vi "Version_2.0_Single_Column_Code.vi"() -> ()   [LabVIEW 2020] (continued)
                            n921 = local write "Valve V6 Open"(FALSE ("Valve V6 Open")) -> ()
                            n922 = local write "Valve V7 Open"(FALSE ("Valve V7 Open")) -> ()
                          }
                          frame #3 {
                            n923 = local read "Apparent Volume\nof Syringe"() -> (w1396:dbl)
                            n924 = local read "Sample Volume \nto be Pumped"() -> (w1399:dbl)
                            n925 = Quotient & Remainder(x=w1399, y=w1396) -> (x-y*floor(x/y)=w1397:dbl, floor(x/y)=w1398:dbl)
                            n926 = for {
                              N: w1398 -> [_]
                              n927 = stacked-sequence {
                                frame #0 {
                                n928 = local read "Sample PickUp \nFlow Rate (ul/min)"() -> (w1402:dbl)
                                n929 = local read "Sample Pumping\nResolution"() -> (w1401:T2)
                                n930 = local read "VISA Refnum in\nfor Pump"() -> (w1404:refnum<visa-resource-name>)
                                n931 = local read "Apparent Volume\nof Syringe"() -> (w1400:dbl)
                                n932 = local read "Volume of Syringe"() -> (w1403:dbl)
                                n933 = call "RPickUp(SubVI).vi"("Volume to be picked up"=w1400, "Volume of Syringe"=w1403, "Resolution of PickUP"=w1401, "PickUp Flow Rate (ul/min)"=w1402, "VISA Refnum in"=w1404) -> ()  [unwired: 6 in, 1 out]
                                }
                                frame #1 {
                                n934 = local read "Stopper that ends \nthe main loops"() -> (w1405:bool)
                                n935 = local read "VISA Refnum in\nfor Pump"() -> (w1406:refnum<visa-resource-name>)
                                n936 = case shown="True" w1405 {
                                frame False {
                                }
                                frame True {
                                n937 = local read "VISA Refnum in\nfor Pump"() -> (w1407:refnum<visa-resource-name>)
                                n938 = call "HardStopCurrentProcess (SubVI).vi"("VISA Refnum in"=w1407) -> ()  [unwired: 11 in]
                                }
                                }
                                n939 = call "ProcessCompletionWaiter (SubVI).vi"("VISA Refnum in"=w1406) -> ()  [unwired: 11 in]
                                }
                                frame #2 {
                                # "Reads the initial Plunger Position for computing the volume dispensed"
                                n940 = local read "VISA Refnum in\nfor Pump"() -> (w1409:refnum<visa-resource-name>)
                                n941 = call "AbsolutePlungerPosition (SubVI).vi"("VISA Refnum in"=w1409) -> ("Plunger Position"=w1408:i32)  [unwired: 10 in]
                                n942 = local write "Initial Plunger Position"(w1408) -> ()
                                }
                                frame #3 {
                                # "Switch to Port-2"
                                # "Port-2 of the pump is conncted to column-1 of chip"
                                n943 = local read "VISA Refnum in\nfor Pump"() -> (w1411:refnum<visa-resource-name>)
                                n944 = call "PortChanger (SubVI).vi"("Port Number"="2", "VISA Refnum in"=w1411) -> ()  [unwired: 10 in]
                                }
                                frame #4 {
                                n945 = local read "Stopper that ends \nthe main loops"() -> (w1412:bool)
                                n946 = local read "VISA Refnum in\nfor Pump"() -> (w1413:refnum<visa-resource-name>)
                                n947 = case shown="True" w1412 {
                                frame False {
                                }
                                frame True {
                                n948 = local read "VISA Refnum in\nfor Pump"() -> (w1414:refnum<visa-resource-name>)
                                n949 = call "HardStopCurrentProcess (SubVI).vi"("VISA Refnum in"=w1414) -> ()  [unwired: 11 in]
                                }
                                }
                                n950 = call "ProcessCompletionWaiter (SubVI).vi"("VISA Refnum in"=w1413) -> ()  [unwired: 11 in]
                                }
                                frame #5 {
                                # "Keeps the AMF valve after column-1 open and valve after column-2 closed"
                                n951 = local read "Sample Dispense\nFlow Rate (ul/min)"() -> (w1418:dbl)
                                n952 = local read "Sample Pumping\nResolution"() -> (w1417:T2)
                                n953 = local read "VISA Refnum in\nfor Pump"() -> (w1420:refnum<visa-resource-name>)
                                n954 = local write "Pause Data Collection"(FALSE ("Pause Data Collection")) -> ()
                                n955 = local read "Volume of Syringe"() -> (w1419:dbl)
                                n956 = call "GoToAbsolutePosition(SubVI).vi"("Absolute Volume Position in Syringe (in ul)"=0.0 ("Volume to be Dispensed"), "Volume of Syringe"=w1419, "Resolution of Pumping"=w1417, "Flow Rate (ul/min)"=w1418, "VISA Refnum in"=w1420) -> ()  [unwired: 6 in, 1 out]
                                }
                                frame #6 {
                                n957 = local read "Sample Pumping\nResolution"() -> (w1422:T2)
                                n958 = local read "VISA Refnum in\nfor Pump"() -> (w1424:refnum<visa-resource-name>)
                                n959 = local read "Initial Plunger Position"() -> (w1423:dbl)
                                n960 = local read "Volume of Syringe"() -> (w1421:dbl)
                                n961 = while {
                                tunnel: w1423 -> [w1431]
                                tunnel: w1424 -> [w1430]
                                tunnel: w1422 -> [w1429]
                                tunnel: w1421 -> [w1428]
                                stop <- w1426 stop-if-true
                                n962 = stacked-sequence {
                                tunnel: w1431 -> [w1438 _]
                                tunnel: w1430 -> [w1437 w1458]
                                tunnel: w1429 -> [w1436 _]
                                tunnel: w1428 -> [w1435 _]
                                tunnel: [_ w1456] -> w1426
                                frame #0 {
                                n963 = call "AbsolutePlungerPosition (SubVI).vi"("VISA Refnum in"=w1437) -> ("Plunger Position"=w1434:i32)  [unwired: 10 in]
                                n964 = case shown="\"Standard Pumping\", Default" w1436 {
                                tunnel: w1438 -> [w1443 w1452]
                                tunnel: w1434 -> [w1444 w1451]
                                tunnel: [w1442 w1449] -> w1433
                                tunnel: w1435 -> [w1441 w1450]
                                frame "Standard Pumping", Default {
                                n965 = Subtract(x=w1443, y=w1444) -> (x-y=w1440:dbl)
                                n966 = Absolute Value(x=w1440) -> (abs(x)=w1439:dbl)
                                n967 = Multiply(x=w1439, y=w1441) -> (x*y=w1446:dbl)
                                n968 = Divide(x=w1446, y=3000.0) -> (x/y=w1442:dbl)
                                }
                                frame "High Resolution Pumping" {
                                n969 = Subtract(x=w1452, y=w1451) -> (x-y=w1448:dbl)
                                n970 = Absolute Value(x=w1448) -> (abs(x)=w1447:dbl)
                                n971 = Multiply(x=w1447, y=w1450) -> (x*y=w1454:dbl)
                                n972 = Divide(x=w1454, y=24000.0) -> (x/y=w1449:dbl)
                                }
                                }
                                n973 = local write "Volume being Injected \nin this process"(w1433) -> ()
                                }
                                frame #1 {
                                n974 = call "LSPOneStatus (SubVI).vi"("VISA Refnum in"=w1458) -> ("read buffer"=w1460:string)  [unwired: 10 in]
                                n975 = call <vilib>:"Trim Whitespace.vi"("string"=w1460) -> ("trimmed string"=w1459:string)  [unwired: 1 in]
                                n976 = local read "Stopper that ends \nthe main loops"() -> (w1455:bool)
                                n977 = Equal?(x=w1459, y="/0`\u0003") -> (x = y?=w1457:bool)
                                n978 = Or(x=w1457, y=w1455) -> (x .or. y?=w1456:bool)
                                }
                                }
                                n979 = Wait (ms)(milliseconds to wait=u32 100) -> ()  [unwired: 1 out]
                                n980 = local read "Stopper that ends \nthe main loops"() -> (w1425:bool)
                                n981 = case shown="True" w1425 {
                                frame False {
                                }
                                frame True {
                                n982 = local read "VISA Refnum in\nfor Pump"() -> (w1432:refnum<visa-resource-name>)
                                n983 = call "HardStopCurrentProcess (SubVI).vi"("VISA Refnum in"=w1432) -> ()  [unwired: 11 in]
                                }
                                }
                                }
                                }
                                frame #7 {
                                # "Chnage the pump port back to Sample"
                                n984 = local read "VISA Refnum in\nfor Pump"() -> (w1463:refnum<visa-resource-name>)
                                n985 = local read "Port for \nSample"() -> (w1462:string)
                                n986 = local write "Pause Data Collection"(TRUE ("Pause Data Collection")) -> ()
                                n987 = Wait (ms)(milliseconds to wait=u32 500) -> ()  [unwired: 1 out]
                                n988 = call "PortChanger (SubVI).vi"("Port Number"=w1462, "VISA Refnum in"=w1463) -> ()  [unwired: 10 in]
                                }
                                frame #8 {
                                n989 = local read "VISA Refnum in\nfor Pump"() -> (w1466:refnum<visa-resource-name>)
                                n990 = local write "Volume being Injected \nin this process"(0.0 ("Volume being Injected \nin this process")) -> ()
                                n991 = call "ProcessCompletionWaiter (SubVI).vi"("VISA Refnum in"=w1466) -> ()  [unwired: 11 in]
                                }
                              }
                            }
                            n992 = local write "Reminder of the \nVolume to be \nPumped"(w1397) -> ()
                          }
                          frame #4 {
                            n993 = stacked-sequence {
                              frame #0 {
                                n994 = local read "Sample PickUp \nFlow Rate (ul/min)"() -> (w1470:dbl)
                                n995 = local read "Sample Pumping\nResolution"() -> (w1469:T2)
                                n996 = local read "VISA Refnum in\nfor Pump"() -> (w1472:refnum<visa-resource-name>)
                                n997 = local read "Reminder of the \nVolume to be \nPumped"() -> (w1468:dbl)
                                n998 = local read "Volume of Syringe"() -> (w1471:dbl)
                                n999 = call "RPickUp(SubVI).vi"("Volume to be picked up"=w1468, "Volume of Syringe"=w1471, "Resolution of PickUP"=w1469, "PickUp Flow Rate (ul/min)"=w1470, "VISA Refnum in"=w1472) -> ()  [unwired: 6 in, 1 out]
                              }
                              frame #1 {
                                n1000 = local read "Stopper that ends \nthe main loops"() -> (w1473:bool)
                                n1001 = local read "VISA Refnum in\nfor Pump"() -> (w1474:refnum<visa-resource-name>)
                                n1002 = case shown="True" w1473 {
                                frame False {
                                }
                                frame True {
                                n1003 = local read "VISA Refnum in\nfor Pump"() -> (w1475:refnum<visa-resource-name>)
                                n1004 = call "HardStopCurrentProcess (SubVI).vi"("VISA Refnum in"=w1475) -> ()  [unwired: 11 in]
                                }
                                }
                                n1005 = call "ProcessCompletionWaiter (SubVI).vi"("VISA Refnum in"=w1474) -> ()  [unwired: 11 in]
                              }
                              frame #2 {
                                # "Reads the initial Plunger Position for computing the volume dispensed"
                                n1006 = local read "VISA Refnum in\nfor Pump"() -> (w1477:refnum<visa-resource-name>)
                                n1007 = call "AbsolutePlungerPosition (SubVI).vi"("VISA Refnum in"=w1477) -> ("Plunger Position"=w1476:i32)  [unwired: 10 in]
                                n1008 = local write "Initial Plunger Position"(w1476) -> ()
                              }
                              frame #3 {
                                # "Switch to Port-2"
                                # "Port-2 of the pump is conncted to column-1 of chip"
                                n1009 = local read "VISA Refnum in\nfor Pump"() -> (w1479:refnum<visa-resource-name>)
                                n1010 = call "PortChanger (SubVI).vi"("Port Number"="2", "VISA Refnum in"=w1479) -> ()  [unwired: 10 in]
                              }
                              frame #4 {
                                n1011 = local read "Stopper that ends \nthe main loops"() -> (w1480:bool)
                                n1012 = local read "VISA Refnum in\nfor Pump"() -> (w1481:refnum<visa-resource-name>)
                                n1013 = case shown="True" w1480 {
                                frame False {
                                }
                                frame True {
                                n1014 = local read "VISA Refnum in\nfor Pump"() -> (w1482:refnum<visa-resource-name>)
                                n1015 = call "HardStopCurrentProcess (SubVI).vi"("VISA Refnum in"=w1482) -> ()  [unwired: 11 in]
                                }
                                }
                                n1016 = call "ProcessCompletionWaiter (SubVI).vi"("VISA Refnum in"=w1481) -> ()  [unwired: 11 in]
                              }
                              frame #5 {
                                # "Keeps the AMF valve after column-1 open and valve after column-2 closed"
                                n1017 = local read "Sample Dispense\nFlow Rate (ul/min)"() -> (w1486:dbl)
                                n1018 = local read "Sample Pumping\nResolution"() -> (w1485:T2)
                                n1019 = local read "VISA Refnum in\nfor Pump"() -> (w1488:refnum<visa-resource-name>)
                                n1020 = local write "Pause Data Collection"(FALSE ("Pause Data Collection")) -> ()
                                n1021 = local read "Volume of Syringe"() -> (w1487:dbl)
                                n1022 = call "GoToAbsolutePosition(SubVI).vi"("Absolute Volume Position in Syringe (in ul)"=0.0 ("Volume to be Dispensed"), "Volume of Syringe"=w1487, "Resolution of Pumping"=w1485, "Flow Rate (ul/min)"=w1486, "VISA Refnum in"=w1488) -> ()  [unwired: 6 in, 1 out]
                              }
                              frame #6 {
                                n1023 = local read "Sample Pumping\nResolution"() -> (w1490:T2)
                                n1024 = local read "VISA Refnum in\nfor Pump"() -> (w1492:refnum<visa-resource-name>)
                                n1025 = local read "Initial Plunger Position"() -> (w1491:dbl)
                                n1026 = local read "Volume of Syringe"() -> (w1489:dbl)
                                n1027 = while {
                                tunnel: w1491 -> [w1499]
                                tunnel: w1492 -> [w1498]
                                tunnel: w1490 -> [w1497]
                                tunnel: w1489 -> [w1496]
                                stop <- w1494 stop-if-true
                                n1028 = stacked-sequence {
                                tunnel: w1499 -> [w1506 _]
                                tunnel: w1498 -> [w1505 w1526]
                                tunnel: w1497 -> [w1504 _]
                                tunnel: w1496 -> [w1503 _]
                                tunnel: [_ w1524] -> w1494
                                frame #0 {
                                n1029 = call "AbsolutePlungerPosition (SubVI).vi"("VISA Refnum in"=w1505) -> ("Plunger Position"=w1502:i32)  [unwired: 10 in]
                                n1030 = case shown="\"Standard Pumping\", Default" w1504 {
                                tunnel: w1506 -> [w1511 w1520]
                                tunnel: w1502 -> [w1512 w1519]
                                tunnel: [w1510 w1517] -> w1501
                                tunnel: w1503 -> [w1509 w1518]
                                frame "Standard Pumping", Default {
                                n1031 = Subtract(x=w1511, y=w1512) -> (x-y=w1508:dbl)
                                n1032 = Absolute Value(x=w1508) -> (abs(x)=w1507:dbl)
                                n1033 = Multiply(x=w1507, y=w1509) -> (x*y=w1514:dbl)
                                n1034 = Divide(x=w1514, y=3000.0) -> (x/y=w1510:dbl)
                                }
                                frame "High Resolution Pumping" {
                                n1035 = Subtract(x=w1520, y=w1519) -> (x-y=w1516:dbl)
                                n1036 = Absolute Value(x=w1516) -> (abs(x)=w1515:dbl)
                                n1037 = Multiply(x=w1515, y=w1518) -> (x*y=w1522:dbl)
                                n1038 = Divide(x=w1522, y=24000.0) -> (x/y=w1517:dbl)
                                }
                                }
                                n1039 = local write "Volume being Injected \nin this process"(w1501) -> ()
                                }
                                frame #1 {
                                n1040 = call "LSPOneStatus (SubVI).vi"("VISA Refnum in"=w1526) -> ("read buffer"=w1528:string)  [unwired: 10 in]
                                n1041 = call <vilib>:"Trim Whitespace.vi"("string"=w1528) -> ("trimmed string"=w1527:string)  [unwired: 1 in]
                                n1042 = local read "Stopper that ends \nthe main loops"() -> (w1523:bool)
                                n1043 = Equal?(x=w1527, y="/0`\u0003") -> (x = y?=w1525:bool)
                                n1044 = Or(x=w1525, y=w1523) -> (x .or. y?=w1524:bool)
                                }
                                }
                                n1045 = Wait (ms)(milliseconds to wait=u32 100) -> ()  [unwired: 1 out]
                                n1046 = local read "Stopper that ends \nthe main loops"() -> (w1493:bool)
                                n1047 = case shown="True" w1493 {
                                frame False {
                                }
                                frame True {
                                n1048 = local read "VISA Refnum in\nfor Pump"() -> (w1500:refnum<visa-resource-name>)
                                n1049 = call "HardStopCurrentProcess (SubVI).vi"("VISA Refnum in"=w1500) -> ()  [unwired: 11 in]
                                }
                                }
                                }
                              }
                              frame #7 {
                                n1050 = local write "Pause Data Collection"(TRUE ("Pause Data Collection")) -> ()
                                n1051 = Wait (ms)(milliseconds to wait=u32 500) -> ()  [unwired: 1 out]
                              }
                              frame #8 {
                                n1052 = local write "Volume being Injected \nin this process"(0.0 ("Volume being Injected \nin this process")) -> ()
                              }
                            }
                          }
                        }
                        n1053 = local write "Equilibriating \nColumn-2"(FALSE ("Equilibriating \nColumn-2")) -> ()
                        n1054 = local write "Affinity On"(TRUE ("Affinity On")) -> ()
                        n1055 = local write "Sample pumping \ninto Column-1"(TRUE ("Sample pumping \ninto Column-1")) -> ()
                      }
                      frame #2 {
                        # "Wash Column-1 with Buffer-A2"
                        n1056 = stacked-sequence {
                          frame #0 {
                            # "Switch to Port-4/6"
                            # "Port-4/6 of pump is connected to Buffer-A2"
                            n1057 = local read "VISA Refnum in\nfor Pump"() -> (w1536:refnum<visa-resource-name>)
                            n1058 = local read "Port for \nA2-Wash"() -> (w1535:string)
                            n1059 = call "PortChanger (SubVI).vi"("Port Number"=w1535, "VISA Refnum in"=w1536) -> ()  [unwired: 10 in]
                          }
                          frame #1 {
                            n1060 = local read "VISA Refnum in\nfor Pump"() -> (w1537:refnum<visa-resource-name>)
                            n1061 = call "ProcessCompletionWaiter (SubVI).vi"("VISA Refnum in"=w1537) -> ()  [unwired: 11 in]
                          }
                          frame #2 {
                            n1062 = local read "VISA Refnum in\nfor Valve"() -> (w1541:refnum<visa-resource-name>)
                            n1063 = local read "External Valve \nOPEN"() -> (w1542:string)
                            n1064 = local write "Valve V3 Open"(FALSE ("Valve V3 Open")) -> ()
                            n1065 = local write "Valve V4 Open"(FALSE ("Valve V4 Open")) -> ()
                            n1066 = local write "Valve V1 Open"(TRUE ("Valve V1 Open")) -> ()
                            n1067 = local write "Valve V2 Open"(TRUE ("Valve V2 Open")) -> ()
                            n1068 = call "PortChanger_Valve (SubVI).vi"("Port Number"=w1542, "VISA Refnum in"=w1541) -> ()  [unwired: 10 in]
                            n1069 = local write "Valve V5 Open"(FALSE ("Valve V5 Open")) -> ()
                            n1070 = local write "Valve V6 Open"(FALSE ("Valve V6 Open")) -> ()
                            n1071 = local write "Valve V7 Open"(FALSE ("Valve V7 Open")) -> ()
                          }
                          frame #3 {
                            n1072 = local read "Buffer-A2 Volume \nto be Pumped"() -> (w1550:dbl)
                            n1073 = local read "Apparent Volume\nof Syringe"() -> (w1547:dbl)
                            n1074 = Quotient & Remainder(x=w1550, y=w1547) -> (x-y*floor(x/y)=w1548:dbl, floor(x/y)=w1549:dbl)
                            n1075 = for {
                              N: w1549 -> [_]
                              n1076 = stacked-sequence {
                                frame #0 {
                                n1077 = local read "Buffer-A2 PickUp \nFlow Rate (ul/min)"() -> (w1553:dbl)
                                n1078 = local read "Buffer-A2 Pumping\nResolution"() -> (w1552:T2)
                                n1079 = local read "VISA Refnum in\nfor Pump"() -> (w1555:refnum<visa-resource-name>)
                                n1080 = local read "Apparent Volume\nof Syringe"() -> (w1551:dbl)
                                n1081 = local read "Volume of Syringe"() -> (w1554:dbl)
                                n1082 = call "RPickUp(SubVI).vi"("Volume to be picked up"=w1551, "Volume of Syringe"=w1554, "Resolution of PickUP"=w1552, "PickUp Flow Rate (ul/min)"=w1553, "VISA Refnum in"=w1555) -> ()  [unwired: 6 in, 1 out]
                                }
                                frame #1 {
                                n1083 = local read "Stopper that ends \nthe main loops"() -> (w1556:bool)
                                n1084 = local read "VISA Refnum in\nfor Pump"() -> (w1557:refnum<visa-resource-name>)
                                n1085 = case shown="True" w1556 {
                                frame False {
                                }
                                frame True {
                                n1086 = local read "VISA Refnum in\nfor Pump"() -> (w1558:refnum<visa-resource-name>)
                                n1087 = call "HardStopCurrentProcess (SubVI).vi"("VISA Refnum in"=w1558) -> ()  [unwired: 11 in]
                                }
                                }
                                n1088 = call "ProcessCompletionWaiter (SubVI).vi"("VISA Refnum in"=w1557) -> ()  [unwired: 11 in]
                                }
                                frame #2 {
                                # "Reads the initial Plunger Position for computing the volume dispensed"
                                n1089 = local read "VISA Refnum in\nfor Pump"() -> (w1560:refnum<visa-resource-name>)
                                n1090 = call "AbsolutePlungerPosition (SubVI).vi"("VISA Refnum in"=w1560) -> ("Plunger Position"=w1559:i32)  [unwired: 10 in]
                                n1091 = local write "Initial Plunger Position"(w1559) -> ()
                                }
                                frame #3 {
                                # "Switch to Port-2"
                                # "Port-2 of the pump is conncted to column-1 of chip"
                                n1092 = local read "VISA Refnum in\nfor Pump"() -> (w1562:refnum<visa-resource-name>)
                                n1093 = call "PortChanger (SubVI).vi"("Port Number"="2", "VISA Refnum in"=w1562) -> ()  [unwired: 10 in]
                                }
                                frame #4 {
                                n1094 = local read "Stopper that ends \nthe main loops"() -> (w1563:bool)
                                n1095 = local read "VISA Refnum in\nfor Pump"() -> (w1564:refnum<visa-resource-name>)
                                n1096 = case shown="True" w1563 {
                                frame False {
                                }
                                frame True {
                                n1097 = local read "VISA Refnum in\nfor Pump"() -> (w1565:refnum<visa-resource-name>)
                                n1098 = call "HardStopCurrentProcess (SubVI).vi"("VISA Refnum in"=w1565) -> ()  [unwired: 11 in]
                                }
                                }
                                n1099 = call "ProcessCompletionWaiter (SubVI).vi"("VISA Refnum in"=w1564) -> ()  [unwired: 11 in]
                                }
                                frame #5 {
                                # "Keeps the AMF valve after column-1 open and valve after column-2 closed"
                                n1100 = local read "Buffer-A2 Dispense\nFlow Rate (ul/min)"() -> (w1569:dbl)
                                n1101 = local read "Buffer-A2 Pumping\nResolution"() -> (w1568:T2)
                                n1102 = local read "VISA Refnum in\nfor Pump"() -> (w1571:refnum<visa-resource-name>)
                                n1103 = local write "Pause Data Collection"(FALSE ("Pause Data Collection")) -> ()
                                n1104 = local read "Volume of Syringe"() -> (w1570:dbl)
                                n1105 = call "GoToAbsolutePosition(SubVI).vi"("Absolute Volume Position in Syringe (in ul)"=0.0 ("Volume to be Dispensed"), "Volume of Syringe"=w1570, "Resolution of Pumping"=w1568, "Flow Rate (ul/min)"=w1569, "VISA Refnum in"=w1571) -> ()  [unwired: 6 in, 1 out]
                                }
                                frame #6 {
                                n1106 = local read "Buffer-A2 Pumping\nResolution"() -> (w1573:T2)
                                n1107 = local read "VISA Refnum in\nfor Pump"() -> (w1575:refnum<visa-resource-name>)
                                n1108 = local read "Initial Plunger Position"() -> (w1574:dbl)
                                n1109 = local read "Volume of Syringe"() -> (w1572:dbl)
                                n1110 = while {
                                tunnel: w1574 -> [w1582]
                                tunnel: w1575 -> [w1581]
                                tunnel: w1573 -> [w1580]
                                tunnel: w1572 -> [w1579]
                                stop <- w1577 stop-if-true
                                n1111 = stacked-sequence {
                                tunnel: w1582 -> [w1589 _]
                                tunnel: w1581 -> [w1588 w1609]
                                tunnel: w1580 -> [w1587 _]
                                tunnel: w1579 -> [w1586 _]
                                tunnel: [_ w1607] -> w1577
                                frame #0 {
                                n1112 = call "AbsolutePlungerPosition (SubVI).vi"("VISA Refnum in"=w1588) -> ("Plunger Position"=w1585:i32)  [unwired: 10 in]
                                n1113 = case shown="\"Standard Pumping\", Default" w1587 {
                                tunnel: w1589 -> [w1594 w1603]
                                tunnel: w1585 -> [w1595 w1602]
                                tunnel: [w1593 w1600] -> w1584
                                tunnel: w1586 -> [w1592 w1601]
                                frame "Standard Pumping", Default {
                                n1114 = Subtract(x=w1594, y=w1595) -> (x-y=w1591:dbl)
                                n1115 = Absolute Value(x=w1591) -> (abs(x)=w1590:dbl)
                                n1116 = Multiply(x=w1590, y=w1592) -> (x*y=w1597:dbl)
                                n1117 = Divide(x=w1597, y=3000.0) -> (x/y=w1593:dbl)
                                }
                                frame "High Resolution Pumping" {
                                n1118 = Subtract(x=w1603, y=w1602) -> (x-y=w1599:dbl)
                                n1119 = Absolute Value(x=w1599) -> (abs(x)=w1598:dbl)
                                n1120 = Multiply(x=w1598, y=w1601) -> (x*y=w1605:dbl)
                                n1121 = Divide(x=w1605, y=24000.0) -> (x/y=w1600:dbl)
                                }
                                }
                                n1122 = local write "Volume being Injected \nin this process"(w1584) -> ()
                                }
                                frame #1 {
                                n1123 = call "LSPOneStatus (SubVI).vi"("VISA Refnum in"=w1609) -> ("read buffer"=w1611:string)  [unwired: 10 in]
                                n1124 = call <vilib>:"Trim Whitespace.vi"("string"=w1611) -> ("trimmed string"=w1610:string)  [unwired: 1 in]
                                n1125 = local read "Stopper that ends \nthe main loops"() -> (w1606:bool)
                                n1126 = Equal?(x=w1610, y="/0`\u0003") -> (x = y?=w1608:bool)
                                n1127 = Or(x=w1608, y=w1606) -> (x .or. y?=w1607:bool)
                                }
                                }
                                n1128 = Wait (ms)(milliseconds to wait=u32 100) -> ()  [unwired: 1 out]
                                n1129 = local read "Stopper that ends \nthe main loops"() -> (w1576:bool)
                                n1130 = case shown="True" w1576 {
                                frame False {
                                }
                                frame True {
                                n1131 = local read "VISA Refnum in\nfor Pump"() -> (w1583:refnum<visa-resource-name>)
                                n1132 = call "HardStopCurrentProcess (SubVI).vi"("VISA Refnum in"=w1583) -> ()  [unwired: 11 in]
                                }
                                }
                                }
                                }
                                frame #7 {
                                # "Change the port back to Buffer-A2"
                                n1133 = local read "VISA Refnum in\nfor Pump"() -> (w1614:refnum<visa-resource-name>)
                                n1134 = local read "Port for \nA2-Wash"() -> (w1613:string)
                                n1135 = local write "Pause Data Collection"(TRUE ("Pause Data Collection")) -> ()
                                n1136 = Wait (ms)(milliseconds to wait=u32 500) -> ()  [unwired: 1 out]
                                n1137 = call "PortChanger (SubVI).vi"("Port Number"=w1613, "VISA Refnum in"=w1614) -> ()  [unwired: 10 in]
                                }
                                frame #8 {
                                n1138 = local read "VISA Refnum in\nfor Pump"() -> (w1617:refnum<visa-resource-name>)
                                n1139 = local write "Volume being Injected \nin this process"(0.0 ("Volume being Injected \nin this process")) -> ()
                                n1140 = call "ProcessCompletionWaiter (SubVI).vi"("VISA Refnum in"=w1617) -> ()  [unwired: 11 in]
                                }
                              }
                            }
                            n1141 = local write "Reminder of the \nVolume to be \nPumped"(w1548) -> ()
                          }
                          frame #4 {
                            n1142 = stacked-sequence {
                              frame #0 {
                                n1143 = local read "Buffer-A2 PickUp \nFlow Rate (ul/min)"() -> (w1621:dbl)
                                n1144 = local read "Buffer-A2 Pumping\nResolution"() -> (w1620:T2)
                                n1145 = local read "VISA Refnum in\nfor Pump"() -> (w1623:refnum<visa-resource-name>)
                                n1146 = local read "Reminder of the \nVolume to be \nPumped"() -> (w1619:dbl)
                                n1147 = local read "Volume of Syringe"() -> (w1622:dbl)
                                n1148 = call "RPickUp(SubVI).vi"("Volume to be picked up"=w1619, "Volume of Syringe"=w1622, "Resolution of PickUP"=w1620, "PickUp Flow Rate (ul/min)"=w1621, "VISA Refnum in"=w1623) -> ()  [unwired: 6 in, 1 out]
                              }
                              frame #1 {
                                n1149 = local read "Stopper that ends \nthe main loops"() -> (w1624:bool)
                                n1150 = local read "VISA Refnum in\nfor Pump"() -> (w1625:refnum<visa-resource-name>)
                                n1151 = case shown="True" w1624 {
                                frame False {
                                }
                                frame True {
                                n1152 = local read "VISA Refnum in\nfor Pump"() -> (w1626:refnum<visa-resource-name>)
                                n1153 = call "HardStopCurrentProcess (SubVI).vi"("VISA Refnum in"=w1626) -> ()  [unwired: 11 in]
                                }
                                }
                                n1154 = call "ProcessCompletionWaiter (SubVI).vi"("VISA Refnum in"=w1625) -> ()  [unwired: 11 in]
                              }
                              frame #2 {
                                # "Reads the initial Plunger Position for computing the volume dispensed"
                                n1155 = local read "VISA Refnum in\nfor Pump"() -> (w1628:refnum<visa-resource-name>)
                                n1156 = call "AbsolutePlungerPosition (SubVI).vi"("VISA Refnum in"=w1628) -> ("Plunger Position"=w1627:i32)  [unwired: 10 in]
                                n1157 = local write "Initial Plunger Position"(w1627) -> ()
                              }
                              frame #3 {
                                # "Switch to Port-2"
                                # "Port-2 of the pump is conncted to column-1 of chip"
                                n1158 = local read "VISA Refnum in\nfor Pump"() -> (w1630:refnum<visa-resource-name>)
                                n1159 = call "PortChanger (SubVI).vi"("Port Number"="2", "VISA Refnum in"=w1630) -> ()  [unwired: 10 in]
                              }
                              frame #4 {
                                n1160 = local read "Stopper that ends \nthe main loops"() -> (w1631:bool)
                                n1161 = local read "VISA Refnum in\nfor Pump"() -> (w1632:refnum<visa-resource-name>)
                                n1162 = case shown="True" w1631 {
                                frame False {
                                }
                                frame True {
                                n1163 = local read "VISA Refnum in\nfor Pump"() -> (w1633:refnum<visa-resource-name>)
                                n1164 = call "HardStopCurrentProcess (SubVI).vi"("VISA Refnum in"=w1633) -> ()  [unwired: 11 in]
                                }
                                }
                                n1165 = call "ProcessCompletionWaiter (SubVI).vi"("VISA Refnum in"=w1632) -> ()  [unwired: 11 in]
                              }
                              frame #5 {
                                # "Keeps the AMF valve after column-1 open and valve after column-2 closed"
                                n1166 = local read "Buffer-A2 Dispense\nFlow Rate (ul/min)"() -> (w1637:dbl)
                                n1167 = local read "Buffer-A2 Pumping\nResolution"() -> (w1636:T2)
                                n1168 = local read "VISA Refnum in\nfor Pump"() -> (w1639:refnum<visa-resource-name>)
                                n1169 = local write "Pause Data Collection"(FALSE ("Pause Data Collection")) -> ()
                                n1170 = local read "Volume of Syringe"() -> (w1638:dbl)
                                n1171 = call "GoToAbsolutePosition(SubVI).vi"("Absolute Volume Position in Syringe (in ul)"=0.0 ("Volume to be Dispensed"), "Volume of Syringe"=w1638, "Resolution of Pumping"=w1636, "Flow Rate (ul/min)"=w1637, "VISA Refnum in"=w1639) -> ()  [unwired: 6 in, 1 out]
                              }
                              frame #6 {
                                n1172 = local read "Buffer-A2 Pumping\nResolution"() -> (w1641:T2)
                                n1173 = local read "VISA Refnum in\nfor Pump"() -> (w1643:refnum<visa-resource-name>)
                                n1174 = local read "Initial Plunger Position"() -> (w1642:dbl)
                                n1175 = local read "Volume of Syringe"() -> (w1640:dbl)
                                n1176 = while {
                                tunnel: w1642 -> [w1650]
                                tunnel: w1643 -> [w1649]
                                tunnel: w1641 -> [w1648]
                                tunnel: w1640 -> [w1647]
                                stop <- w1645 stop-if-true
                                n1177 = stacked-sequence {
                                tunnel: w1650 -> [w1657 _]
                                tunnel: w1649 -> [w1656 w1677]
                                tunnel: w1648 -> [w1655 _]
                                tunnel: w1647 -> [w1654 _]
                                tunnel: [_ w1675] -> w1645
                                frame #0 {
                                n1178 = call "AbsolutePlungerPosition (SubVI).vi"("VISA Refnum in"=w1656) -> ("Plunger Position"=w1653:i32)  [unwired: 10 in]
                                n1179 = case shown="\"Standard Pumping\", Default" w1655 {
                                tunnel: w1657 -> [w1662 w1671]
                                tunnel: w1653 -> [w1663 w1670]
                                tunnel: [w1661 w1668] -> w1652
                                tunnel: w1654 -> [w1660 w1669]
                                frame "Standard Pumping", Default {
                                n1180 = Subtract(x=w1662, y=w1663) -> (x-y=w1659:dbl)
                                n1181 = Absolute Value(x=w1659) -> (abs(x)=w1658:dbl)
                                n1182 = Multiply(x=w1658, y=w1660) -> (x*y=w1665:dbl)
                                n1183 = Divide(x=w1665, y=3000.0) -> (x/y=w1661:dbl)
                                }
                                frame "High Resolution Pumping" {
                                n1184 = Subtract(x=w1671, y=w1670) -> (x-y=w1667:dbl)
                                n1185 = Absolute Value(x=w1667) -> (abs(x)=w1666:dbl)
                                n1186 = Multiply(x=w1666, y=w1669) -> (x*y=w1673:dbl)
                                n1187 = Divide(x=w1673, y=24000.0) -> (x/y=w1668:dbl)
                                }
                                }
                                n1188 = local write "Volume being Injected \nin this process"(w1652) -> ()
                                }
                                frame #1 {
                                n1189 = call "LSPOneStatus (SubVI).vi"("VISA Refnum in"=w1677) -> ("read buffer"=w1679:string)  [unwired: 10 in]
                                n1190 = call <vilib>:"Trim Whitespace.vi"("string"=w1679) -> ("trimmed string"=w1678:string)  [unwired: 1 in]
                                n1191 = local read "Stopper that ends \nthe main loops"() -> (w1674:bool)
                                n1192 = Equal?(x=w1678, y="/0`\u0003") -> (x = y?=w1676:bool)
                                n1193 = Or(x=w1676, y=w1674) -> (x .or. y?=w1675:bool)
                                }
                                }
                                n1194 = Wait (ms)(milliseconds to wait=u32 100) -> ()  [unwired: 1 out]
                                n1195 = local read "Stopper that ends \nthe main loops"() -> (w1644:bool)
                                n1196 = case shown="True" w1644 {
                                frame False {
                                }
                                frame True {
                                n1197 = local read "VISA Refnum in\nfor Pump"() -> (w1651:refnum<visa-resource-name>)
                                n1198 = call "HardStopCurrentProcess (SubVI).vi"("VISA Refnum in"=w1651) -> ()  [unwired: 11 in]
                                }
                                }
                                }
                              }
                              frame #7 {
                                n1199 = local write "Pause Data Collection"(TRUE ("Pause Data Collection")) -> ()
                                n1200 = Wait (ms)(milliseconds to wait=u32 500) -> ()  [unwired: 1 out]
                              }
                              frame #8 {
                                n1201 = local write "Volume being Injected \nin this process"(0.0 ("Volume being Injected \nin this process")) -> ()
                                n1202 = local write "Start the Process"(FALSE ("Start the Process")) -> ()
                              }
                            }
                          }
                        }
                        n1203 = local write "Sample pumping \ninto Column-1"(FALSE ("Sample pumping \ninto Column-1")) -> ()
                        n1204 = local write "Washing Column-1"(TRUE ("Washing Column-1")) -> ()
                      }
                      frame #3 {
                        # "Connecting Buffer-C with port-5, cleaning the tubing with Buffer-C1, and washing the Column-2 to get rid of spill out from wash steps of column-1"
                        n1205 = stacked-sequence {
                          frame #0 {
                            # "Switch to Port-5"
                            # "Port-5 of pump is connected to Buffer-C1"
                            n1206 = local read "VISA Refnum in\nfor Pump"() -> (w1688:refnum<visa-resource-name>)
                            n1207 = local read "Port for \nC1-Equilibriation"() -> (w1687:string)
                            n1208 = call "PortChanger (SubVI).vi"("Port Number"=w1687, "VISA Refnum in"=w1688) -> ()  [unwired: 10 in]
                          }
                          frame #1 {
                            n1209 = local read "VISA Refnum in\nfor Pump"() -> (w1689:refnum<visa-resource-name>)
                            n1210 = call "ProcessCompletionWaiter (SubVI).vi"("VISA Refnum in"=w1689) -> ()  [unwired: 11 in]
                          }
                          frame #2 {
                            # "Wash the inside of the pump valve"
                            n1211 = local read "n"() -> (w1690:i32)
                            n1212 = for {
                              N: w1690 -> [_]
                              n1213 = stacked-sequence {
                                frame #0 {
                                n1214 = local read "Buffer-A2 Pumping\nResolution"() -> (w1693:T2)
                                n1215 = local read "VISA Refnum in\nfor Pump"() -> (w1695:refnum<visa-resource-name>)
                                n1216 = local read "V-S"() -> (w1691:dbl)
                                n1217 = local read "Volume of Syringe"() -> (w1694:dbl)
                                n1218 = call "RPickUp(SubVI).vi"("Volume to be picked up"=w1691, "Volume of Syringe"=w1694, "Resolution of PickUP"=w1693, "PickUp Flow Rate (ul/min)"=150.0, "VISA Refnum in"=w1695) -> ()  [unwired: 6 in, 1 out]
                                }
                                frame #1 {
                                n1219 = local read "Stopper that ends \nthe main loops"() -> (w1696:bool)
                                n1220 = local read "VISA Refnum in\nfor Pump"() -> (w1697:refnum<visa-resource-name>)
                                n1221 = case shown="True" w1696 {
                                frame False {
                                }
                                frame True {
                                n1222 = local read "VISA Refnum in\nfor Pump"() -> (w1698:refnum<visa-resource-name>)
                                n1223 = call "HardStopCurrentProcess (SubVI).vi"("VISA Refnum in"=w1698) -> ()  [unwired: 11 in]
                                }
                                }
                                n1224 = call "ProcessCompletionWaiter (SubVI).vi"("VISA Refnum in"=w1697) -> ()  [unwired: 11 in]
                                }
                                frame #2 {
                                # "Switch to Port-1"
                                # "Port-1 of the pump is conncted to waste"
                                n1225 = local read "VISA Refnum in\nfor Pump"() -> (w1700:refnum<visa-resource-name>)
                                n1226 = call "PortChanger (SubVI).vi"("Port Number"="1", "VISA Refnum in"=w1700) -> ()  [unwired: 10 in]
                                }
                                frame #3 {
                                n1227 = local read "Stopper that ends \nthe main loops"() -> (w1701:bool)
                                n1228 = local read "VISA Refnum in\nfor Pump"() -> (w1702:refnum<visa-resource-name>)
                                n1229 = case shown="True" w1701 {
                                frame False {
                                }
                                frame True {
                                n1230 = local read "VISA Refnum in\nfor Pump"() -> (w1703:refnum<visa-resource-name>)
                                n1231 = call "HardStopCurrentProcess (SubVI).vi"("VISA Refnum in"=w1703) -> ()  [unwired: 11 in]
                                }
                                }
                                n1232 = call "ProcessCompletionWaiter (SubVI).vi"("VISA Refnum in"=w1702) -> ()  [unwired: 11 in]
                                }
                                frame #4 {
                                n1233 = local read "Buffer-A2 Pumping\nResolution"() -> (w1706:T2)
                                n1234 = local read "VISA Refnum in\nfor Pump"() -> (w1708:refnum<visa-resource-name>)
                                n1235 = local read "Volume of Syringe"() -> (w1707:dbl)
                                n1236 = call "GoToAbsolutePosition(SubVI).vi"("Absolute Volume Position in Syringe (in ul)"=0.0 ("Volume to be Dispensed"), "Volume of Syringe"=w1707, "Resolution of Pumping"=w1706, "Flow Rate (ul/min)"=150.0, "VISA Refnum in"=w1708) -> ()  [unwired: 6 in, 1 out]
                                }
                                frame #5 {
                                n1237 = local read "VISA Refnum in\nfor Pump"() -> (w1709:refnum<visa-resource-name>)
                                n1238 = call "ProcessCompletionWaiter (SubVI).vi"("VISA Refnum in"=w1709) -> ()  [unwired: 11 in]
                                }
                                frame #6 {
                                # "Change the port back to Buffer-C1"
                                n1239 = local read "VISA Refnum in\nfor Pump"() -> (w1711:refnum<visa-resource-name>)
                                n1240 = local read "Port for \nC1-Equilibriation"() -> (w1710:string)
                                n1241 = call "PortChanger (SubVI).vi"("Port Number"=w1710, "VISA Refnum in"=w1711) -> ()  [unwired: 10 in]
                                }
                                frame #7 {
                                n1242 = local read "VISA Refnum in\nfor Pump"() -> (w1712:refnum<visa-resource-name>)
                                n1243 = call "ProcessCompletionWaiter (SubVI).vi"("VISA Refnum in"=w1712) -> ()  [unwired: 11 in]
                                }
                              }
                            }
                          }
                          frame #3 {
                            # "Wash the pathway between column-2 and column-1 on chip"
                            n1244 = local read "n"() -> (w1713:i32)
                            n1245 = for {
                              N: w1713 -> [_]
                              n1246 = stacked-sequence {
                                frame #0 {
                                n1247 = local read "Buffer-A2 Pumping\nResolution"() -> (w1716:T2)
                                n1248 = local read "VISA Refnum in\nfor Pump"() -> (w1718:refnum<visa-resource-name>)
                                n1249 = local read "V-S"() -> (w1714:dbl)
                                n1250 = local read "Volume of Syringe"() -> (w1717:dbl)
                                n1251 = call "RPickUp(SubVI).vi"("Volume to be picked up"=w1714, "Volume of Syringe"=w1717, "Resolution of PickUP"=w1716, "PickUp Flow Rate (ul/min)"=150.0, "VISA Refnum in"=w1718) -> ()  [unwired: 6 in, 1 out]
                                }
                                frame #1 {
                                n1252 = local read "Stopper that ends \nthe main loops"() -> (w1719:bool)
                                n1253 = local read "VISA Refnum in\nfor Pump"() -> (w1720:refnum<visa-resource-name>)
                                n1254 = case shown="True" w1719 {
                                frame False {
                                }
                                frame True {
                                n1255 = local read "VISA Refnum in\nfor Pump"() -> (w1721:refnum<visa-resource-name>)
                                n1256 = call "HardStopCurrentProcess (SubVI).vi"("VISA Refnum in"=w1721) -> ()  [unwired: 11 in]
                                }
                                }
                                n1257 = call "ProcessCompletionWaiter (SubVI).vi"("VISA Refnum in"=w1720) -> ()  [unwired: 11 in]
                                }
                                frame #2 {
                                # "Switch to Port-10"
                                # "Port-10 of the pump is conncted to column-2"
                                n1258 = local read "VISA Refnum in\nfor Pump"() -> (w1723:refnum<visa-resource-name>)
                                n1259 = call "PortChanger (SubVI).vi"("Port Number"="10", "VISA Refnum in"=w1723) -> ()  [unwired: 10 in]
                                }
                                frame #3 {
                                n1260 = local read "Stopper that ends \nthe main loops"() -> (w1724:bool)
                                n1261 = local read "VISA Refnum in\nfor Pump"() -> (w1725:refnum<visa-resource-name>)
                                n1262 = case shown="True" w1724 {
                                frame False {
                                }
                                frame True {
                                n1263 = local read "VISA Refnum in\nfor Pump"() -> (w1726:refnum<visa-resource-name>)
                                n1264 = call "HardStopCurrentProcess (SubVI).vi"("VISA Refnum in"=w1726) -> ()  [unwired: 11 in]
                                }
                                }
                                n1265 = call "ProcessCompletionWaiter (SubVI).vi"("VISA Refnum in"=w1725) -> ()  [unwired: 11 in]
                                }
                                frame #4 {
                                n1266 = local read "Buffer-A2 Pumping\nResolution"() -> (w1735:T2)
                                n1267 = local read "VISA Refnum in\nfor Pump"() -> (w1737:refnum<visa-resource-name>)
                                n1268 = local read "f"() -> (w1727:dbl)
                                n1269 = local read "Volume of Syringe"() -> (w1736:dbl)
                                n1270 = call "GoToAbsolutePosition(SubVI).vi"("Absolute Volume Position in Syringe (in ul)"=0.0 ("Volume to be Dispensed"), "Volume of Syringe"=w1736, "Resolution of Pumping"=w1735, "Flow Rate (ul/min)"=w1727, "VISA Refnum in"=w1737) -> ()  [unwired: 6 in, 1 out]
                                n1271 = local read "VISA Refnum in\nfor Valve"() -> (w1729:refnum<visa-resource-name>)
                                n1272 = local read "External Valve \nOPEN"() -> (w1728:string)
                                n1273 = local write "Valve V2 Open"(TRUE ("Valve V2 Open")) -> ()
                                n1274 = local write "Valve V1 Open"(FALSE ("Valve V1 Open")) -> ()
                                n1275 = local write "Valve V4 Open"(FALSE ("Valve V4 Open")) -> ()
                                n1276 = local write "Valve V3 Open"(TRUE ("Valve V3 Open")) -> ()
                                n1277 = call "PortChanger_Valve (SubVI).vi"("Port Number"=w1728, "VISA Refnum in"=w1729) -> ()  [unwired: 10 in]
                                }
                                frame #5 {
                                n1278 = local read "VISA Refnum in\nfor Pump"() -> (w1738:refnum<visa-resource-name>)
                                n1279 = call "ProcessCompletionWaiter (SubVI).vi"("VISA Refnum in"=w1738) -> ()  [unwired: 11 in]
                                }
                                frame #6 {
                                # "Change the port back to Buffer-C1"
                                n1280 = local read "VISA Refnum in\nfor Pump"() -> (w1740:refnum<visa-resource-name>)
                                n1281 = local read "Port for \nC1-Equilibriation"() -> (w1739:string)
                                n1282 = call "PortChanger (SubVI).vi"("Port Number"=w1739, "VISA Refnum in"=w1740) -> ()  [unwired: 10 in]
                                }
                                frame #7 {
                                n1283 = local read "VISA Refnum in\nfor Pump"() -> (w1741:refnum<visa-resource-name>)
                                n1284 = call "ProcessCompletionWaiter (SubVI).vi"("VISA Refnum in"=w1741) -> ()  [unwired: 11 in]
                                }
                              }
                            }
                          }
                          frame #4 {
                            # "Washes the SEC column"
                            n1285 = local read "Apparent Volume\nof Syringe"() -> (w1744:dbl)
                            n1286 = local read "c"() -> (w1745:dbl)
                            n1287 = Quotient & Remainder(x=w1745, y=w1744) -> (x-y*floor(x/y)=w1743:dbl, floor(x/y)=w1742:dbl)
                            n1288 = for {
                              N: w1742 -> [_]
                              n1289 = stacked-sequence {
                                frame #0 {
                                n1290 = local read "Buffer-A2 Pumping\nResolution"() -> (w1748:T2)
                                n1291 = local read "VISA Refnum in\nfor Pump"() -> (w1750:refnum<visa-resource-name>)
                                n1292 = local read "Apparent Volume\nof Syringe"() -> (w1746:dbl)
                                n1293 = local read "Volume of Syringe"() -> (w1749:dbl)
                                n1294 = call "RPickUp(SubVI).vi"("Volume to be picked up"=w1746, "Volume of Syringe"=w1749, "Resolution of PickUP"=w1748, "PickUp Flow Rate (ul/min)"=150.0, "VISA Refnum in"=w1750) -> ()  [unwired: 6 in, 1 out]
                                }
                                frame #1 {
                                n1295 = local read "Stopper that ends \nthe main loops"() -> (w1751:bool)
                                n1296 = local read "VISA Refnum in\nfor Pump"() -> (w1752:refnum<visa-resource-name>)
                                n1297 = case shown="True" w1751 {
                                frame False {
                                }
                                frame True {
                                n1298 = local read "VISA Refnum in\nfor Pump"() -> (w1753:refnum<visa-resource-name>)
                                n1299 = call "HardStopCurrentProcess (SubVI).vi"("VISA Refnum in"=w1753) -> ()  [unwired: 11 in]
                                }
                                }
                                n1300 = call "ProcessCompletionWaiter (SubVI).vi"("VISA Refnum in"=w1752) -> ()  [unwired: 11 in]
                                }
                                frame #2 {
                                # "Switch to Port-10"
                                # "Port-10 of the pump is conncted to column-2 of chip"
                                n1301 = local read "VISA Refnum in\nfor Pump"() -> (w1755:refnum<visa-resource-name>)
                                n1302 = call "PortChanger (SubVI).vi"("Port Number"="10", "VISA Refnum in"=w1755) -> ()  [unwired: 10 in]
                                }
                                frame #3 {
                                n1303 = local read "Stopper that ends \nthe main loops"() -> (w1756:bool)
                                n1304 = local read "VISA Refnum in\nfor Pump"() -> (w1757:refnum<visa-resource-name>)
                                n1305 = case shown="True" w1756 {
                                frame False {
                                }
                                frame True {
                                n1306 = local read "VISA Refnum in\nfor Pump"() -> (w1758:refnum<visa-resource-name>)
                                n1307 = call "HardStopCurrentProcess (SubVI).vi"("VISA Refnum in"=w1758) -> ()  [unwired: 11 in]
                                }
                                }
                                n1308 = call "ProcessCompletionWaiter (SubVI).vi"("VISA Refnum in"=w1757) -> ()  [unwired: 11 in]
                                }
                                frame #4 {
                                # "Keeps the AMF valve after column-1 open and valve after column-2 closed"
                                n1309 = local read "Buffer-A2 Pumping\nResolution"() -> (w1770:T2)
                                n1310 = local read "VISA Refnum in\nfor Pump"() -> (w1772:refnum<visa-resource-name>)
                                n1311 = local read "f"() -> (w1762:dbl)
                                n1312 = local write "Valve V3 Open"(FALSE ("Valve V3 Open")) -> ()
                                n1313 = local write "Valve V2 Open"(FALSE ("Valve V2 Open")) -> ()
                                n1314 = local write "Valve V4 Open"(TRUE ("Valve V4 Open")) -> ()
                                n1315 = local write "Valve V1 Open"(FALSE ("Valve V1 Open")) -> ()
                                n1316 = local read "Volume of Syringe"() -> (w1771:dbl)
                                n1317 = call "GoToAbsolutePosition(SubVI).vi"("Absolute Volume Position in Syringe (in ul)"=0.0 ("Volume to be Dispensed"), "Volume of Syringe"=w1771, "Resolution of Pumping"=w1770, "Flow Rate (ul/min)"=w1762, "VISA Refnum in"=w1772) -> ()  [unwired: 6 in, 1 out]
                                n1318 = local read "VISA Refnum in\nfor Valve"() -> (w1767:refnum<visa-resource-name>)
                                n1319 = local read "External Valve \nCLOSED"() -> (w1763:string)
                                n1320 = local write "Valve V5 Open"(TRUE ("Valve V5 Open")) -> ()
                                n1321 = local write "Valve V6 Open"(FALSE ("Valve V6 Open")) -> ()
                                n1322 = local write "Valve V7 Open"(TRUE ("Valve V7 Open")) -> ()
                                n1323 = call "PortChanger_Valve (SubVI).vi"("Port Number"=w1763, "VISA Refnum in"=w1767) -> ()  [unwired: 10 in]
                                }
                                frame #5 {
                                n1324 = local read "VISA Refnum in\nfor Pump"() -> (w1773:refnum<visa-resource-name>)
                                n1325 = call "ProcessCompletionWaiter (SubVI).vi"("VISA Refnum in"=w1773) -> ()  [unwired: 11 in]
                                }
                                frame #6 {
                                # "Change the port back to Buffer-C1"
                                n1326 = local read "VISA Refnum in\nfor Pump"() -> (w1775:refnum<visa-resource-name>)
                                n1327 = local read "Port for \nC1-Equilibriation"() -> (w1774:string)
                                n1328 = call "PortChanger (SubVI).vi"("Port Number"=w1774, "VISA Refnum in"=w1775) -> ()  [unwired: 10 in]
                                }
                                frame #7 {
                                n1329 = local read "VISA Refnum in\nfor Pump"() -> (w1776:refnum<visa-resource-name>)
                                n1330 = call "ProcessCompletionWaiter (SubVI).vi"("VISA Refnum in"=w1776) -> ()  [unwired: 11 in]
                                }
                              }
                            }
                            n1331 = local write "Reminder of the \nVolume to be \nPumped"(w1743) -> ()
                          }
                          frame #5 {
                            # "Washes the SEC column"
                            n1332 = stacked-sequence {
                              frame #0 {
                                n1333 = local read "Buffer-A2 Pumping\nResolution"() -> (w1779:T2)
                                n1334 = local read "VISA Refnum in\nfor Pump"() -> (w1781:refnum<visa-resource-name>)
                                n1335 = local read "Reminder of the \nVolume to be \nPumped"() -> (w1777:dbl)
                                n1336 = local read "Volume of Syringe"() -> (w1780:dbl)
                                n1337 = call "RPickUp(SubVI).vi"("Volume to be picked up"=w1777, "Volume of Syringe"=w1780, "Resolution of PickUP"=w1779, "PickUp Flow Rate (ul/min)"=150.0, "VISA Refnum in"=w1781) -> ()  [unwired: 6 in, 1 out]
                              }
                              frame #1 {
                                n1338 = local read "Stopper that ends \nthe main loops"() -> (w1782:bool)
                                n1339 = local read "VISA Refnum in\nfor Pump"() -> (w1783:refnum<visa-resource-name>)
                                n1340 = case shown="True" w1782 {
                                frame False {
                                }
                                frame True {
                                n1341 = local read "VISA Refnum in\nfor Pump"() -> (w1784:refnum<visa-resource-name>)
                                n1342 = call "HardStopCurrentProcess (SubVI).vi"("VISA Refnum in"=w1784) -> ()  [unwired: 11 in]
                                }
                                }
                                n1343 = call "ProcessCompletionWaiter (SubVI).vi"("VISA Refnum in"=w1783) -> ()  [unwired: 11 in]
                              }
                              frame #2 {
                                # "Switch to Port-10"
                                # "Port-10 of the pump is conncted to column-2 of chip"
                                n1344 = local read "VISA Refnum in\nfor Pump"() -> (w1786:refnum<visa-resource-name>)
                                n1345 = call "PortChanger (SubVI).vi"("Port Number"="10", "VISA Refnum in"=w1786) -> ()  [unwired: 10 in]
                              }
                              frame #3 {
                                n1346 = local read "Stopper that ends \nthe main loops"() -> (w1787:bool)
                                n1347 = local read "VISA Refnum in\nfor Pump"() -> (w1788:refnum<visa-resource-name>)
                                n1348 = case shown="True" w1787 {
                                frame False {
                                }
                                frame True {
                                n1349 = local read "VISA Refnum in\nfor Pump"() -> (w1789:refnum<visa-resource-name>)
                                n1350 = call "HardStopCurrentProcess (SubVI).vi"("VISA Refnum in"=w1789) -> ()  [unwired: 11 in]
                                }
                                }
                                n1351 = call "ProcessCompletionWaiter (SubVI).vi"("VISA Refnum in"=w1788) -> ()  [unwired: 11 in]
                              }
                              frame #4 {
                                n1352 = local read "Buffer-A2 Pumping\nResolution"() -> (w1801:T2)
                                n1353 = local read "VISA Refnum in\nfor Pump"() -> (w1803:refnum<visa-resource-name>)
                                n1354 = local read "f"() -> (w1793:dbl)
                                n1355 = local read "Volume of Syringe"() -> (w1802:dbl)
                                n1356 = call "GoToAbsolutePosition(SubVI).vi"("Absolute Volume Position in Syringe (in ul)"=0.0 ("Volume to be Dispensed"), "Volume of Syringe"=w1802, "Resolution of Pumping"=w1801, "Flow Rate (ul/min)"=w1793, "VISA Refnum in"=w1803) -> ()  [unwired: 6 in, 1 out]
                                n1357 = local write "Valve V3 Open"(FALSE ("Valve V3 Open")) -> ()
                                n1358 = local write "Valve V2 Open"(FALSE ("Valve V2 Open")) -> ()
                                n1359 = local write "Valve V1 Open"(FALSE ("Valve V1 Open")) -> ()
                                n1360 = local write "Valve V4 Open"(TRUE ("Valve V4 Open")) -> ()
                                n1361 = local read "VISA Refnum in\nfor Valve"() -> (w1798:refnum<visa-resource-name>)
                                n1362 = local read "External Valve \nCLOSED"() -> (w1794:string)
                                n1363 = local write "Valve V6 Open"(TRUE ("Valve V6 Open")) -> ()
                                n1364 = local write "Valve V5 Open"(TRUE ("Valve V5 Open")) -> ()
                                n1365 = local write "Valve V7 Open"(TRUE ("Valve V7 Open")) -> ()
                                n1366 = call "PortChanger_Valve (SubVI).vi"("Port Number"=w1794, "VISA Refnum in"=w1798) -> ()  [unwired: 10 in]
                              }
                              frame #5 {
                                n1367 = local read "VISA Refnum in\nfor Pump"() -> (w1804:refnum<visa-resource-name>)
                                n1368 = call "ProcessCompletionWaiter (SubVI).vi"("VISA Refnum in"=w1804) -> ()  [unwired: 11 in]
                              }
                            }
                          }
                        }
                        n1369 = local write "Washing Column-1"(FALSE ("Washing Column-1")) -> ()
                        n1370 = local write "Washing Column-2"(TRUE ("Washing Column-2")) -> ()
                      }
                      frame #4 {
                        # "Elute Column-1, Divert Sample into Column-2, Elute column-2 and Divert the sample onto Grid"
                        n1371 = stacked-sequence {
                          frame #0 {
                            # "Switch to Port-7"
                            # "Port-7 of pump is connected to Buffer-B"
                            n1372 = local write "Washing Column-2"(FALSE ("Washing Column-2")) -> ()
                            n1373 = local read "VISA Refnum in\nfor Pump"() -> (w1809:refnum<visa-resource-name>)
                            n1374 = local read "Port for \nB-Elution"() -> (w1807:string)
                            n1375 = local write "Affinity Elution On"(TRUE ("Affinity Elution On")) -> ()
                            n1376 = call "PortChanger (SubVI).vi"("Port Number"=w1807, "VISA Refnum in"=w1809) -> ()  [unwired: 10 in]
                            n1377 = local write "Elution of Column-1"(TRUE ("Elution of Column-1")) -> ()
                          }
                          frame #1 {
                            n1378 = local read "VISA Refnum in\nfor Pump"() -> (w1810:refnum<visa-resource-name>)
                            n1379 = call "ProcessCompletionWaiter (SubVI).vi"("VISA Refnum in"=w1810) -> ()  [unwired: 11 in]
                          }
                          frame #2 {
                            # "If Yes, it will clean the elution buffer from port-5 tubing a bit more"
                            n1380 = local read "Clean the \nBuffer-B tubing"() -> (w1811:bool)
                            n1381 = case shown="True" w1811 {
                              frame False {
                                n1382 = stacked-sequence {
                                frame #0 {
                                n1383 = local read "Buffer-B Pumping\nResolution"() -> (w1814:T2)
                                n1384 = local read "VISA Refnum in\nfor Pump"() -> (w1816:refnum<visa-resource-name>)
                                n1385 = local read "V-S"() -> (w1813:dbl)
                                n1386 = local read "Volume of Syringe"() -> (w1815:dbl)
                                n1387 = call "RPickUp(SubVI).vi"("Volume to be picked up"=w1813, "Volume of Syringe"=w1815, "Resolution of PickUP"=w1814, "PickUp Flow Rate (ul/min)"=150.0, "VISA Refnum in"=w1816) -> ()  [unwired: 6 in, 1 out]
                                }
                                frame #1 {
                                n1388 = local read "Stopper that ends \nthe main loops"() -> (w1817:bool)
                                n1389 = local read "VISA Refnum in\nfor Pump"() -> (w1818:refnum<visa-resource-name>)
                                n1390 = case shown="True" w1817 {
                                frame False {
                                }
                                frame True {
                                n1391 = local read "VISA Refnum in\nfor Pump"() -> (w1819:refnum<visa-resource-name>)
                                n1392 = call "HardStopCurrentProcess (SubVI).vi"("VISA Refnum in"=w1819) -> ()  [unwired: 11 in]
                                }
                                }
                                n1393 = call "ProcessCompletionWaiter (SubVI).vi"("VISA Refnum in"=w1818) -> ()  [unwired: 11 in]
                                }
                                frame #2 {
                                n1394 = local read "VISA Refnum in\nfor Pump"() -> (w1821:refnum<visa-resource-name>)
                                n1395 = call "PortChanger (SubVI).vi"("Port Number"="1", "VISA Refnum in"=w1821) -> ()  [unwired: 10 in]
                                }
                                frame #3 {
                                n1396 = local read "Stopper that ends \nthe main loops"() -> (w1822:bool)
                                n1397 = local read "VISA Refnum in\nfor Pump"() -> (w1823:refnum<visa-resource-name>)
                                n1398 = case shown="True" w1822 {
                                frame False {
                                }
                                frame True {
                                n1399 = local read "VISA Refnum in\nfor Pump"() -> (w1824:refnum<visa-resource-name>)
                                n1400 = call "HardStopCurrentProcess (SubVI).vi"("VISA Refnum in"=w1824) -> ()  [unwired: 11 in]
                                }
                                }
                                n1401 = call "ProcessCompletionWaiter (SubVI).vi"("VISA Refnum in"=w1823) -> ()  [unwired: 11 in]
                                }
                                frame #4 {
                                n1402 = local read "VISA Refnum in\nfor Pump"() -> (w1829:refnum<visa-resource-name>)
                                n1403 = local read "Volume of Syringe"() -> (w1826:dbl)
                                n1404 = call "GoToAbsolutePosition(SubVI).vi"("Absolute Volume Position in Syringe (in ul)"=0.0, "Volume of Syringe"=w1826, "Resolution of Pumping"=T2."Standard Pumping", "Flow Rate (ul/min)"=150.0, "VISA Refnum in"=w1829) -> ()  [unwired: 6 in, 1 out]
                                }
                                frame #5 {
                                n1405 = local read "Stopper that ends \nthe main loops"() -> (w1830:bool)
                                n1406 = local read "VISA Refnum in\nfor Pump"() -> (w1831:refnum<visa-resource-name>)
                                n1407 = case shown="True" w1830 {
                                frame False {
                                }
                                frame True {
                                n1408 = local read "VISA Refnum in\nfor Pump"() -> (w1832:refnum<visa-resource-name>)
                                n1409 = call "HardStopCurrentProcess (SubVI).vi"("VISA Refnum in"=w1832) -> ()  [unwired: 11 in]
                                }
                                }
                                n1410 = call "ProcessCompletionWaiter (SubVI).vi"("VISA Refnum in"=w1831) -> ()  [unwired: 11 in]
                                }
                                }
                              }
                              frame True {
                                n1411 = for {
                                N: 2 -> [_]
                                n1412 = stacked-sequence {
                                frame #0 {
                                n1413 = local read "Buffer-B Pumping\nResolution"() -> (w1836:T2)
                                n1414 = local read "VISA Refnum in\nfor Pump"() -> (w1838:refnum<visa-resource-name>)
                                n1415 = local read "Apparent Volume\nof Syringe"() -> (w1835:dbl)
                                n1416 = local read "Volume of Syringe"() -> (w1837:dbl)
                                n1417 = call "RPickUp(SubVI).vi"("Volume to be picked up"=w1835, "Volume of Syringe"=w1837, "Resolution of PickUP"=w1836, "PickUp Flow Rate (ul/min)"=150.0, "VISA Refnum in"=w1838) -> ()  [unwired: 6 in, 1 out]
                                }
                                frame #1 {
                                n1418 = local read "Stopper that ends \nthe main loops"() -> (w1839:bool)
                                n1419 = local read "VISA Refnum in\nfor Pump"() -> (w1840:refnum<visa-resource-name>)
                                n1420 = case shown="True" w1839 {
                                frame False {
                                }
                                frame True {
                                n1421 = local read "VISA Refnum in\nfor Pump"() -> (w1841:refnum<visa-resource-name>)
                                n1422 = call "HardStopCurrentProcess (SubVI).vi"("VISA Refnum in"=w1841) -> ()  [unwired: 11 in]
                                }
                                }
                                n1423 = call "ProcessCompletionWaiter (SubVI).vi"("VISA Refnum in"=w1840) -> ()  [unwired: 11 in]
                                }
                                frame #2 {
                                n1424 = local read "VISA Refnum in\nfor Pump"() -> (w1843:refnum<visa-resource-name>)
                                n1425 = call "PortChanger (SubVI).vi"("Port Number"="1", "VISA Refnum in"=w1843) -> ()  [unwired: 10 in]
                                }
                                frame #3 {
                                n1426 = local read "Stopper that ends \nthe main loops"() -> (w1844:bool)
                                n1427 = local read "VISA Refnum in\nfor Pump"() -> (w1845:refnum<visa-resource-name>)
                                n1428 = case shown="True" w1844 {
                                frame False {
                                }
                                frame True {
                                n1429 = local read "VISA Refnum in\nfor Pump"() -> (w1846:refnum<visa-resource-name>)
                                n1430 = call "HardStopCurrentProcess (SubVI).vi"("VISA Refnum in"=w1846) -> ()  [unwired: 11 in]
                                }
                                }
                                n1431 = call "ProcessCompletionWaiter (SubVI).vi"("VISA Refnum in"=w1845) -> ()  [unwired: 11 in]
                                }
                                frame #4 {
                                n1432 = local read "VISA Refnum in\nfor Pump"() -> (w1851:refnum<visa-resource-name>)
                                n1433 = local read "Volume of Syringe"() -> (w1848:dbl)
                                n1434 = call "GoToAbsolutePosition(SubVI).vi"("Absolute Volume Position in Syringe (in ul)"=0.0, "Volume of Syringe"=w1848, "Resolution of Pumping"=T2."Standard Pumping", "Flow Rate (ul/min)"=150.0, "VISA Refnum in"=w1851) -> ()  [unwired: 6 in, 1 out]
                                }
                                frame #5 {
                                n1435 = local read "Stopper that ends \nthe main loops"() -> (w1852:bool)
